vi "Data Viewer.vi"() -> ()   [LabVIEW 2018]
uses:
  Type/_Data.ctl
  <vilib>/Analysis/8numeric.llb/1D Numeric Integration.vi
  <vilib>/printing/ReportDocExtensions.llb/Append Front Panel Image to Report (path).vi
  <vilib>/Utility/NIReport.llb/NI_report.lvclass
  <vilib>/Utility/NIReport.llb/NI_ReportGenerationCore.lvlib
  <vilib>/Analysis/NI_AALPro.lvlib
  <vilib>/Analysis/NI_AALBase.lvlib
panel:
  out "File Name":string
  in  "Export 3":bool
  in  "Export 2":bool
  in  "Export":bool
  in  "Clear Last":bool
  in  "X scale to S":bool
  in  "Clear Offset":bool
  in  "Manual Offset":dbl format="%0.2f"
  in  "Subtract Manual":bool
  in  "Subtract File":bool
  in  "Subtract Mean":bool
  out "Mean":dbl format="%0.2f"
  out "Standard Deviation":dbl format="%0.2f"
  in  "Avg 4":bool caption="Avg"
  in  "Log 4":bool caption="Log"
  in  "CPS 4":bool caption="CPS"
  in  "Avg 3":bool caption="Avg"
  in  "Log 3":bool caption="Log"
  in  "CPS 3":bool caption="CPS"
  in  "Clear":bool
  in  "Add Overlay":bool
  out "Overlays":cluster{"X":sgl[], "Y":sgl[]}[](graph) caption="C:\\Users\\Tyler Doodeman\\Desktop\\April 5, 2018\\GC-C6\\722-GC-C6-5uL.isd; TIC=0; T=0mS"
  out "Integral":dbl format="%0.2f"
  out "TIC VS Time":cluster{"X":sgl[], "Y":sgl[]}(graph) caption="D:\\ProgrammsEI\\Sample#1 18_10_15_04_45PM.isd"
  out "XIC":cluster{"X":sgl[], "Y":sgl[]}(graph) caption="D:\\ProgrammsEI\\Sample#1 18_10_15_04_45PM.isd"
  in  "MR#":i32=1 caption="MR #"
  in  "Expt#":i32=1 caption="Expt #"
  in  "Scan#":i32=1 caption="Scan #"
  in  "Avg":bool
  in  "Log":bool
  in  "CPS":bool
  out "Spectrum":cluster{"X":sgl[], "Y":sgl[]}(graph) caption="D:\\ProgrammsEI\\Sample#1 18_10_15_04_45PM.isd; TIC=1; T=0mS"
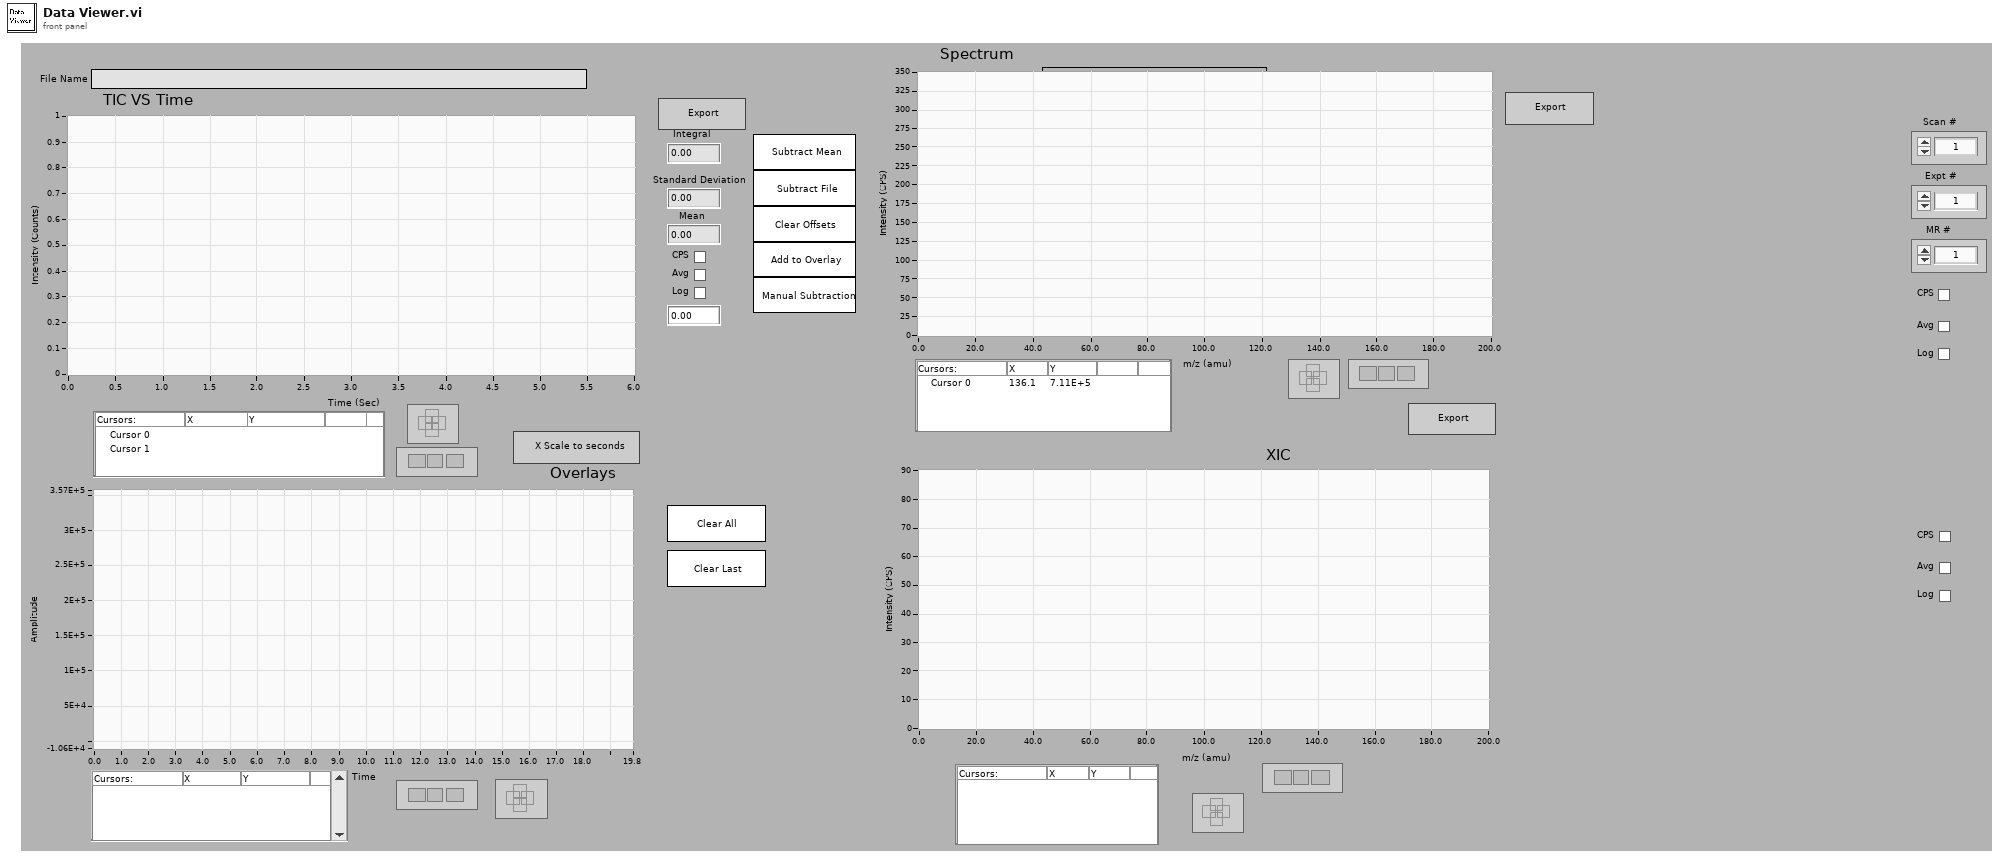
[diagram p1: front panel]
types:
  T1 = typedef "_Data.ctl" = cluster{"X":dbl[], "Y":dbl[], "Dwell Time (mS)":dbl, "X Title":string, "Time (s)":dbl, "TIC":u32, "# of Scans":i32, "Path":path, "ScanType":i32}
  T2 = cluster{"Spectrum Data":T1, "Spectrum":refnum<vi>, "TIC VS Time":refnum<vi>, "Path":path, "TIC Spectrum":refnum<vi>, "TIC VS Time Offset":dbl, "Overlay Offset":dbl, "XIC Data":T1, "Offset":dbl, "File Offset":dbl[], "Overlay Data":cluster{"X":sgl[], "Y":sgl[]}[], "TIC Spectrum":T1}
  T3 = enum32{"existing file", "new file", "new or existing file", "existing dir", "new dir", "new or existing dir", "existing file (use LLBs)", "new file (use LLBs)", "new or existing file (use LLBs)", "new or existing file or directory (use LLBs)"}
  T4 = enum16{"Standard Report", "HTML", "Word", "Excel"}
  T5 = typedef "imagedata.ctl" = cluster{"image type":i32, "image depth":i32, "image":u8[], "mask":u8[], "colors":u32[], "Rectangle":cluster{"left":i16, "top":i16, "right":i16, "bottom":i16}}
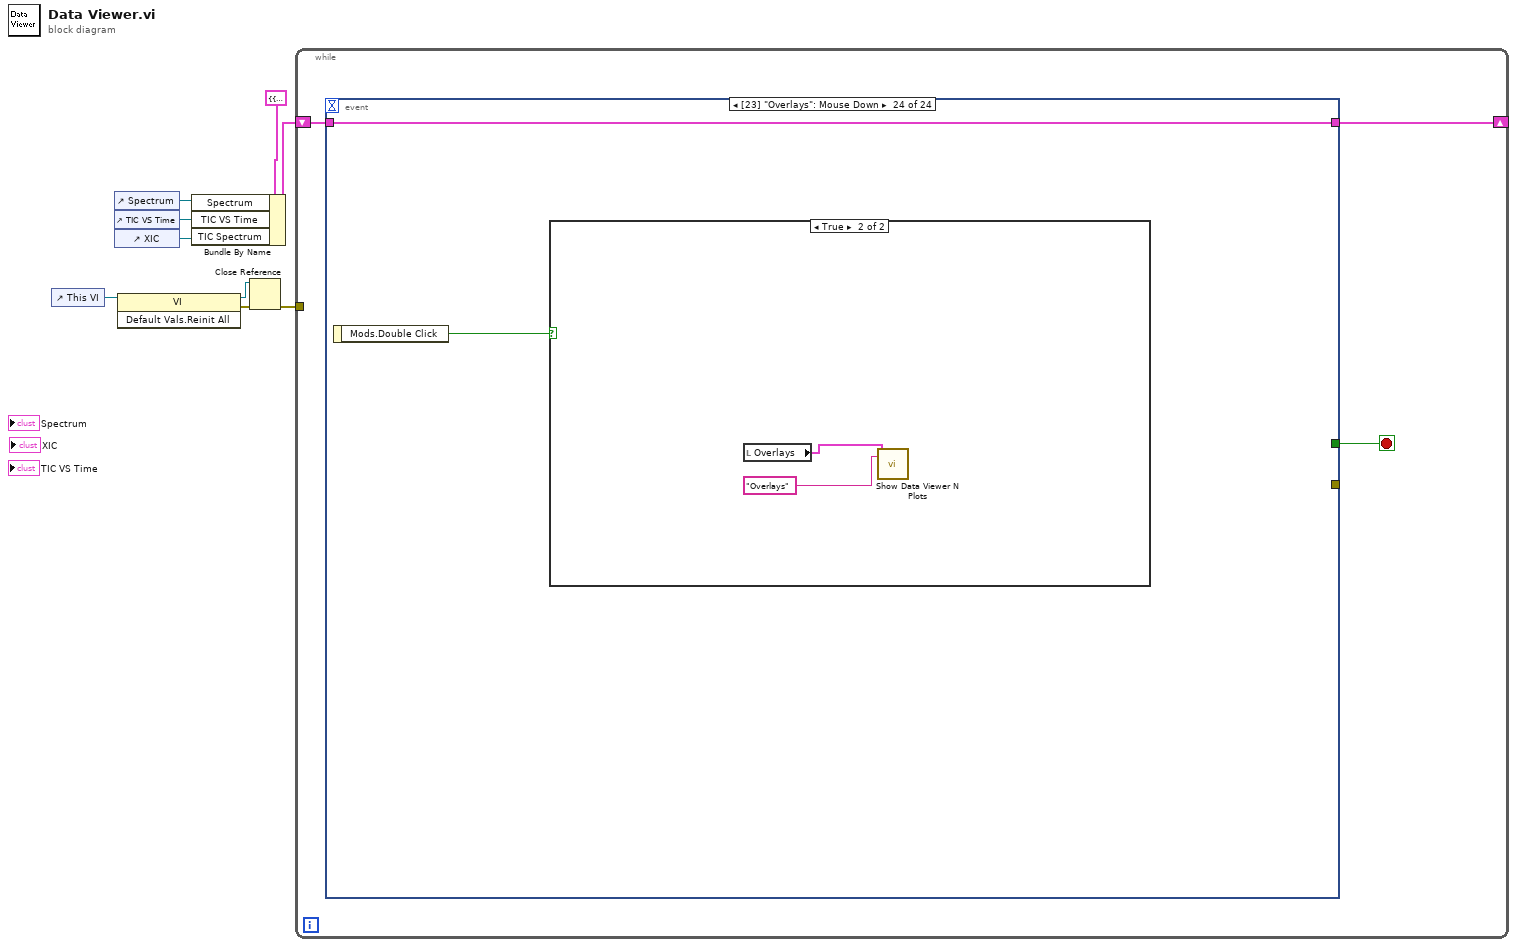
[diagram p0: block diagram]
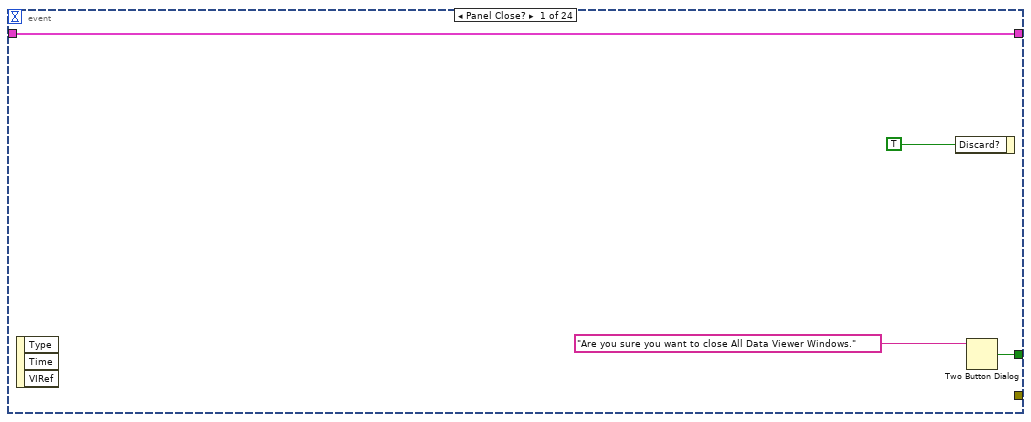
[diagram p2: hidden frame]
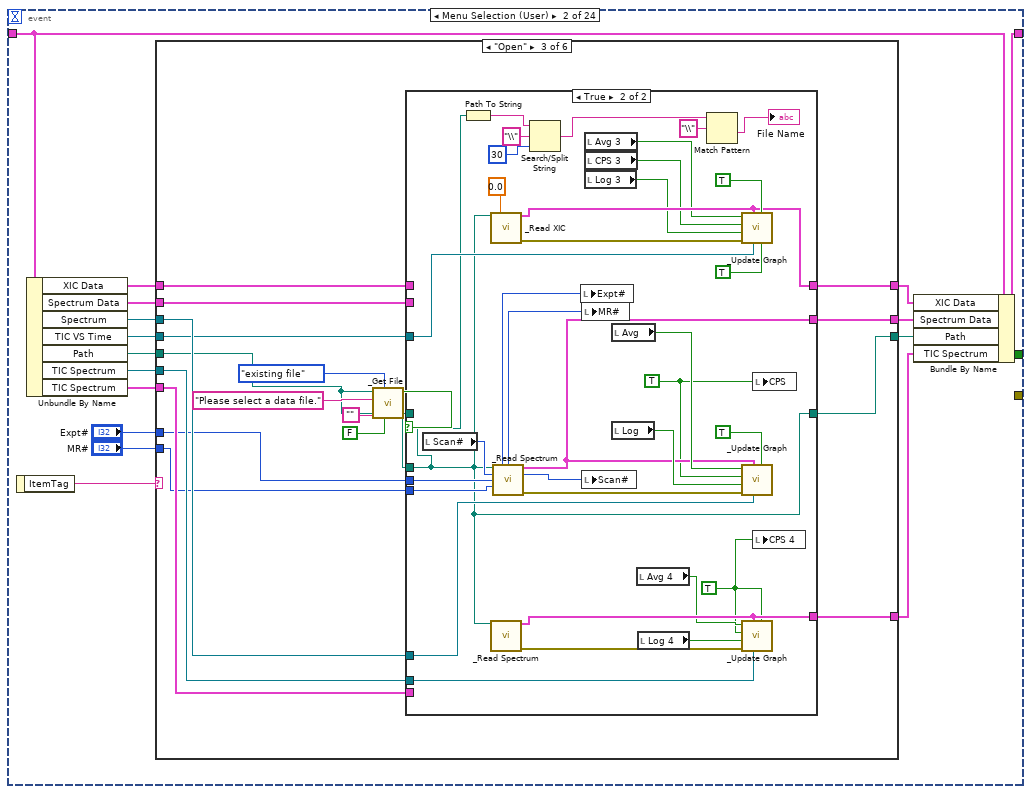
[diagram p3: hidden frame]
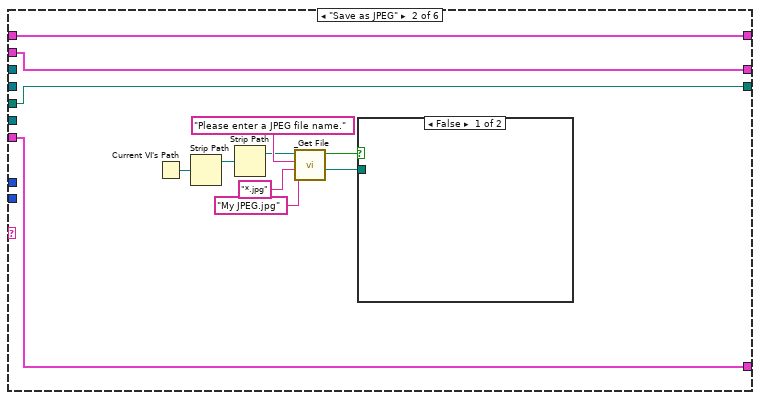
[diagram p5: hidden frame]
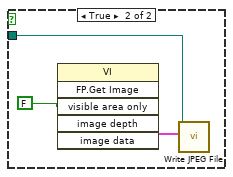
[diagram p6: hidden frame]
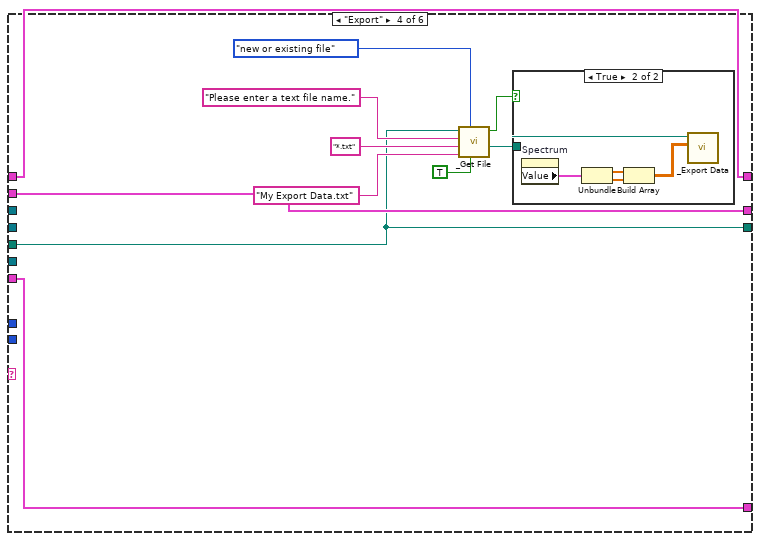
[diagram p8: hidden frame]
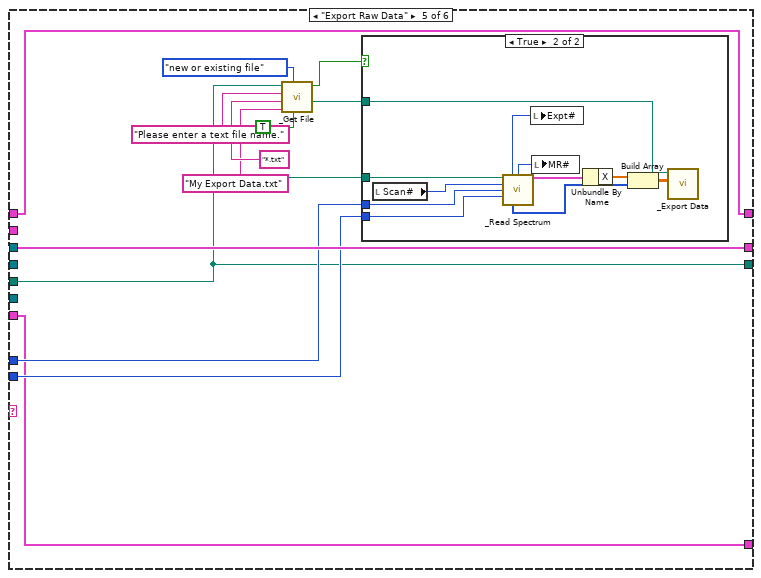
[diagram p10: hidden frame]
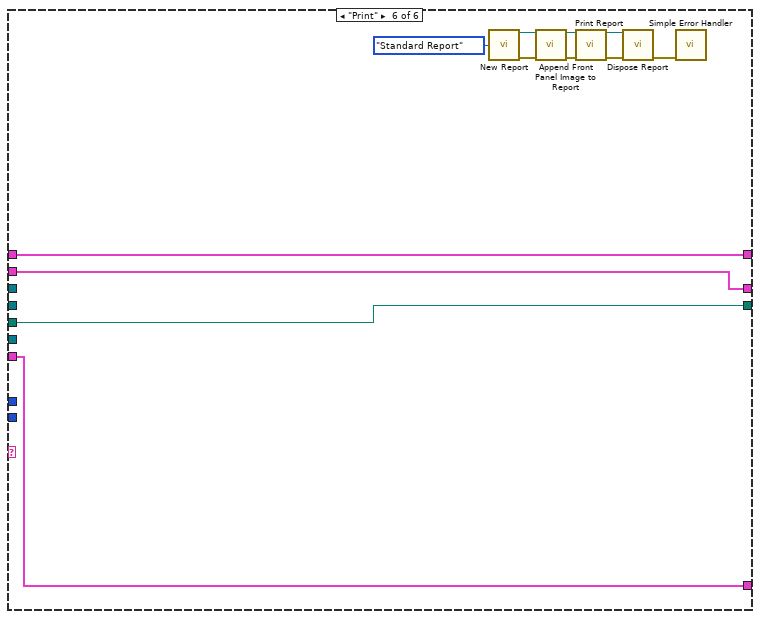
[diagram p12: hidden frame]
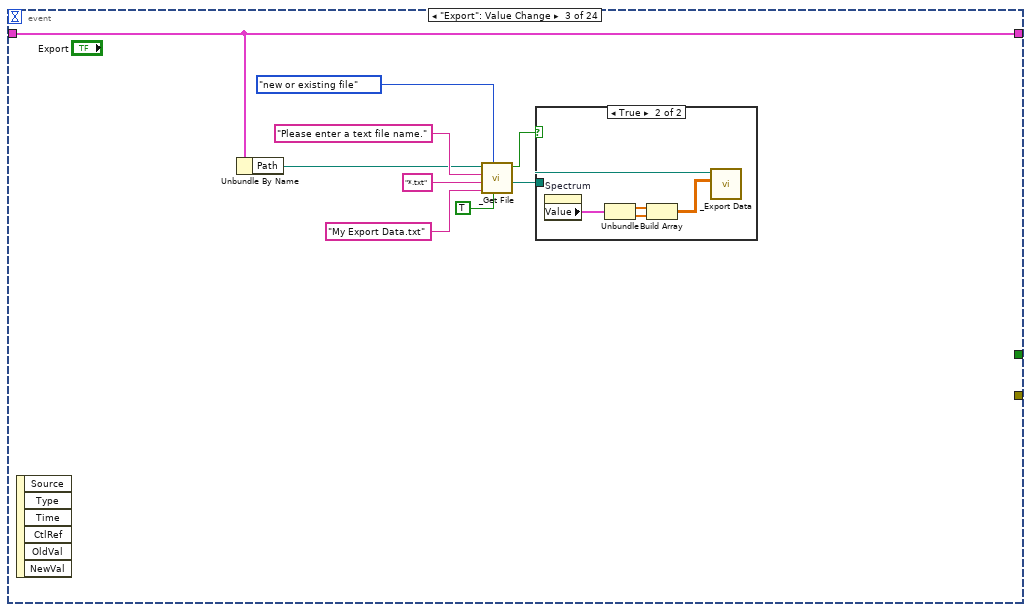
[diagram p13: hidden frame]
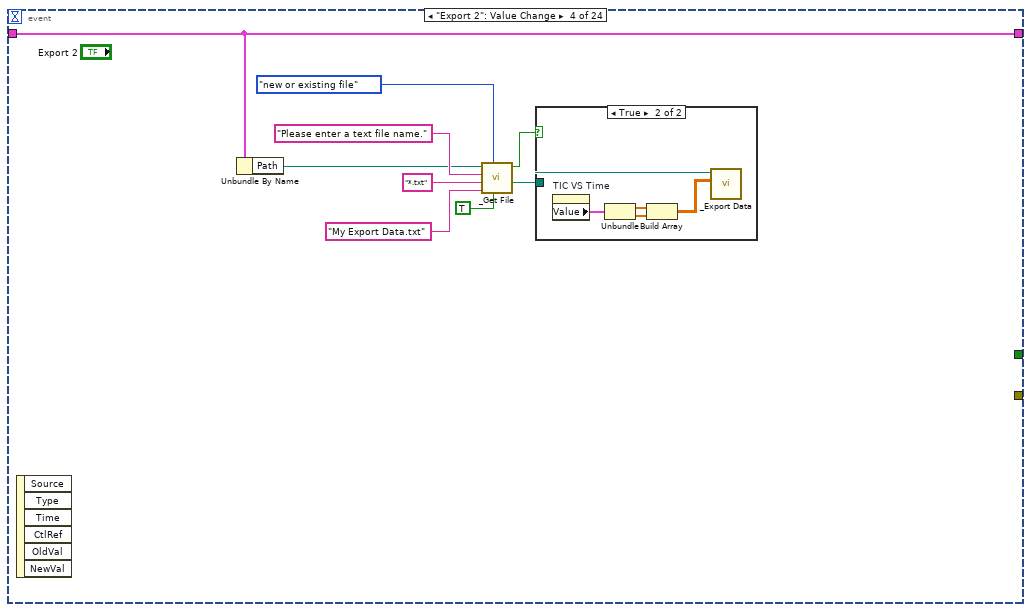
[diagram p15: hidden frame]
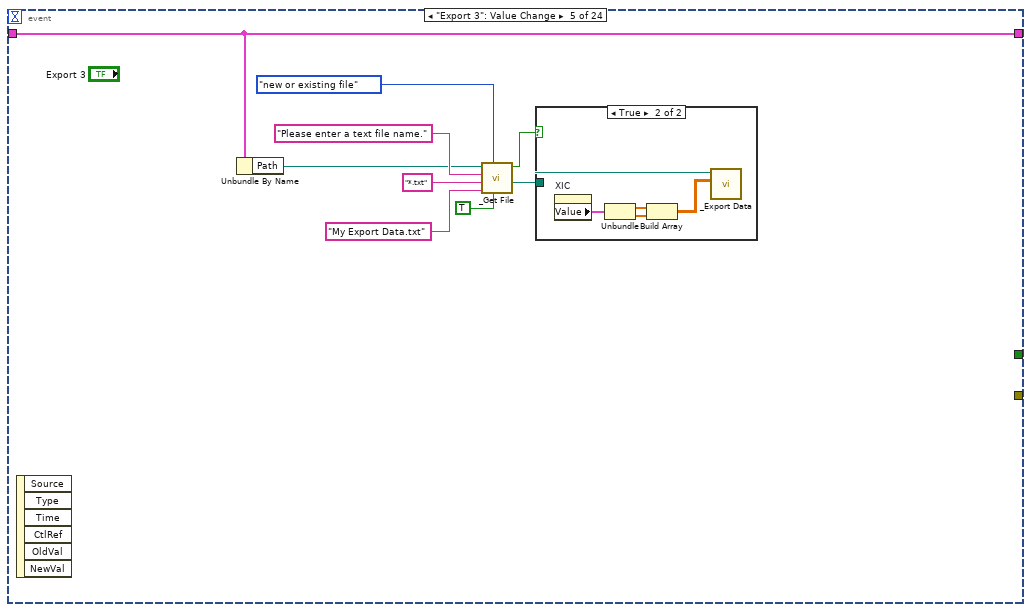
[diagram p17: hidden frame]
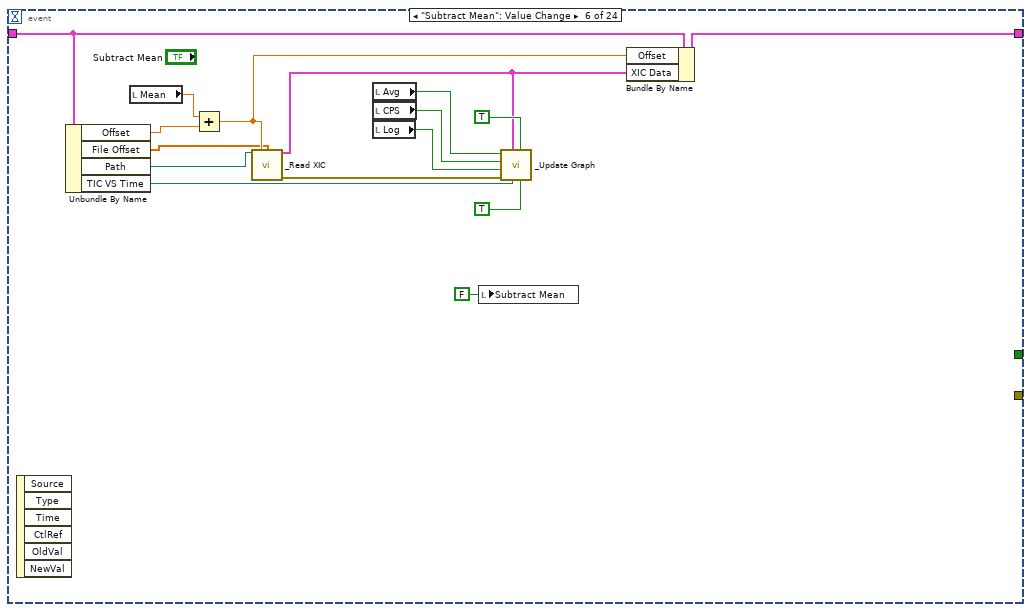
[diagram p19: hidden frame]
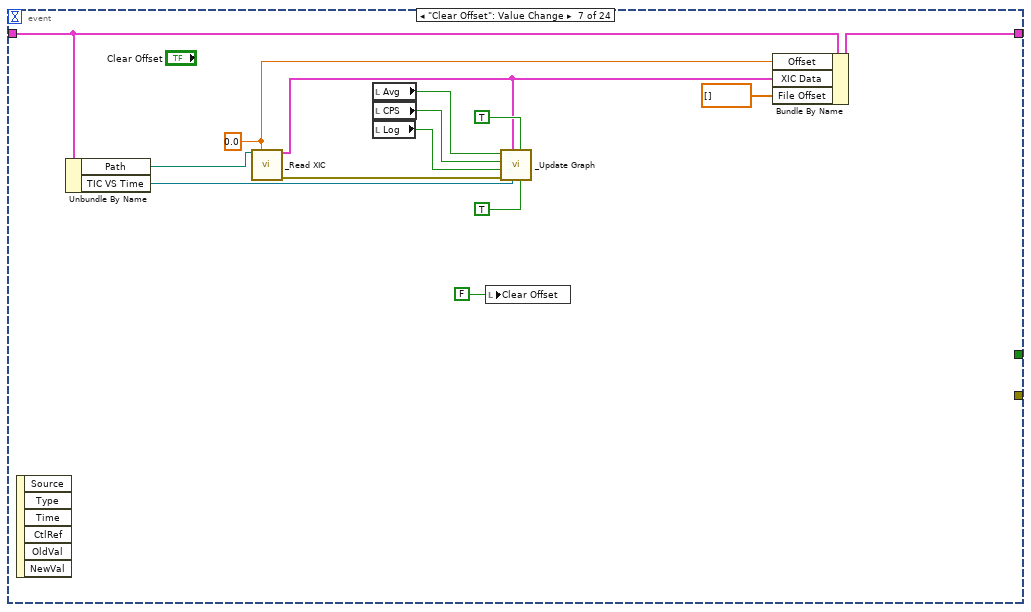
[diagram p20: hidden frame]
diagram:
  n1 = control-ref of="This VI"() -> (w4:refnum<vi>)
  n2 = control-ref of="Spectrum"() -> (w7:refnum<vi>)
  n3 = control-ref of="TIC VS Time"() -> (w6:refnum<vi>)
  n4 = control-ref of="XIC"() -> (w5:refnum<vi>)
  n5 = invoke class="VI" method="Default Vals.Reinit All"(reference=w4) -> (reference out=w2:refnum<vi>, error out=w3:errorcluster)  [unwired: 2 in, 1 out]
  n6 = Bundle By Name(cluster=T2 {"Spectrum Data"={"X"=[], "Y"=[], "Dwell Time (mS)"=0.0, "X Title"="", "Time (s)"=0.0, "TIC"=0, "# of Scans"=0, "Path"=path "", "ScanType"=0}, "Spectrum"=refnum, "TIC VS Time"=refnum, "Path"=path "", "TIC Spectrum"=refnum, "TIC VS Time Offset"=0.0, "Overlay Offset"=0.0, "XIC Data"={"X"=[], "Y"=[], "Dwell Time (mS)"=10.0, "X Title"="", "Time (s)"=0.0, "TIC"=0, "# of Scans"=133, "Path"=path "", "ScanType"=1}, "Offset"=0.0, "File Offset"=[], "Overlay Data"=[], "TIC Spectrum"={"X"=[], "Y"=[], "Dwell Time (mS)"=10.0, "X Title"="", "Time (s)"=0.0, "TIC"=0, "# of Scans"=133, "Path"=path "", "ScanType"=1}}, "Spectrum"=w7, "TIC VS Time"=w6, "TIC Spectrum"=w5) -> (w8:T2)
  n7 = Close Reference(reference=w2, error in (no error)=w3) -> (error out=w1:errorcluster)
  n8 = while {
    shift-right: [w10] -> _
    shift-left: w8 -> [w11]
    tunnel: w1 -> [_]
    stop <- w12 stop-if-true
    n9 = event shown="[23] \"Overlays\": Mouse Down" {
      selector: _ -> [_ _ _ _ _ _ _ _ _ _ _ _ _ _ _ _ _ _ _ _ _ _ _ _]
      dyn-events: _ -> [_ _ _ _ _ _ _ _ _ _ _ _ _ _ _ _ _ _ _ _ _ _ _ _]
      timeout: _ -> [_ _ _ _ _ _ _ _ _ _ _ _ _ _ _ _ _ _ _ _ _ _ _ _]
      tunnel: [w14 _ _ _ _ _ _ _ _ _ _ _ _ _ _ _ _ _ _ _ _ _ _ _] -> w12
      tunnel: w11 -> [w13 w26 w163 w177 w191 w213 w227 w243 w261 w283 w291 w299 w310 w318 w326 w345 w386 w399 w401 w405 w409 w414 w419 w424]
      tunnel: [w13 w25 w163 w177 w191 w210 w224 w240 w259 w281 w290 w299 w309 w318 w326 w344 w388 w399 w401 w405 w409 w414 w419 w424] -> w10
      tunnel: [_ _ _ _ _ _ _ _ _ _ w284 _ _ _ _ _ _ _ _ _ _ _ _ _] -> _
      event Panel Close? {
        n10 = event-data() -> ()  [unwired: 4 out]
        n11 = event-data("Discard?"=TRUE) -> ()  [unwired: 1 in, 1 out]
        n12 = Two Button Dialog(message="Are you sure you want to close All Data Viewer Windows.") -> (T button?=w14:bool)  [unwired: 2 out]
      }
      event Menu Selection (User) {
        n13 = event-data() -> ("ItemTag"=w32:string)  [unwired: 1 out]
        n14 = Unbundle By Name(w26) -> ("XIC Data"=w19:T1, "Spectrum Data"=w29:T1, "Spectrum"=w28:refnum<vi>, "TIC VS Time"=w27:refnum<vi>, "Path"=w22:path, "TIC Spectrum"=w21:refnum<vi>, "TIC Spectrum"=w17:T1)
        n15 = case shown="\"Open\"" w32 {
          tunnel: w29 -> [w36 w37 w66 w113 w131 w161]
          tunnel: [w36 w37 w65 w113 w131 w161] -> w24
          tunnel: w28 -> [_ _ w64 _ _ _]
          tunnel: "Expt#" -> [_ _ w53 _ w130 _]
          tunnel: "MR#" -> [_ _ w52 _ w129 _]
          tunnel: w27 -> [_ _ w62 _ _ _]
          tunnel: [w35 w48 w60 w112 w128 w152] -> w23
          tunnel: w22 -> [w35 w48 w59 w112 w128 w152]
          tunnel: w21 -> [_ _ w58 _ _ _]
          tunnel: [w34 w47 w57 w111 w127 w151] -> w20
          tunnel: w19 -> [w34 w47 w56 w111 w127 w151]
          tunnel: [w33 w46 w55 w110 w126 w150] -> w18
          tunnel: w17 -> [w33 w46 w54 w110 w126 w150]
          frame Default {
          }
          frame "Save as JPEG" {
            n16 = Current VI's Path() -> (path=w38:path)
            n17 = Strip Path(path=w38) -> (stripped path=w39:path)  [unwired: 1 out]
            n18 = Strip Path(path=w39) -> (stripped path=w40:path)  [unwired: 1 out]
            n19 = call "_Get File.vi"("default name"="My JPEG.jpg", "extension (isd)"="*.jpg", "prompt"="Please enter a JPEG file name.", "Start Path"=w40) -> ("Seleted File"=w45:path, "Succeeded"=w44:bool)  [unwired: 2 in, 2 out]
            n20 = case shown="False" w44 {
              tunnel: w45 -> [_ w49]
              frame False {
              }
              frame True {
                n21 = invoke class="VI" method="FP.Get Image"("visible area only"=FALSE ("Visible Area Only")) -> ("image data"=w50:T5)  [unwired: 5 in, 5 out]
                n22 = call <vilib>:"Write JPEG File.vi"("image data"=w50, "path to JPEG file"=w49) -> ()  [unwired: 1 in, 9 out]
              }
            }
          }
          frame "Open" {
            n23 = call "_Get File.vi"("For Write (T)"=FALSE, "select mode (new or existing)"=T3."existing file", "default name"="", "prompt"="Please select a data file.", "Start Path"=w59) -> ("Seleted File"=w61:path, "Succeeded"=w67:bool)  [unwired: 1 in, 2 out]
            n24 = case shown="True" w67 {
              tunnel: w61 -> [_ w88]
              tunnel: w66 -> [w74 _]
              tunnel: [w74 w105] -> w65
              tunnel: w64 -> [_ w104]
              tunnel: w62 -> [_ w96]
              tunnel: [w73 w88] -> w60
              tunnel: w59 -> [w73 _]
              tunnel: w58 -> [_ w95]
              tunnel: [w72 w93] -> w57
              tunnel: w56 -> [w72 _]
              tunnel: [w71 w92] -> w55
              tunnel: w54 -> [w71 _]
              tunnel: w53 -> [_ w91]
              tunnel: w52 -> [_ w90]
              frame False {
              }
              frame True {
                w87 = TRUE ("CPS")
                w82 = TRUE ("Auto Scale")
                n25 = local read "Scan#"() -> (w89:i32)
                n26 = Path To String(path=w88) -> (string=w80:string)
                n27 = call "_Read XIC.vi"("file path"=w88, "Offset"=0.0) -> ("Data"=w93:T1, "error out"=w99:errorcluster)  [unwired: 4 in, 8 out]
                n28 = call "_Read Spectrum.vi"("file path"=w88) -> ("Data"=w92:T1, "error out"=w97:errorcluster)  [unwired: 5 in, 8 out]
                n29 = call "_Read Spectrum.vi"("file path"=w88, "Scan# (1-based)"=w89, "Expt# (1-based)"=w91, "MR# (1-based)"=w90) -> ("Expt# Out"=w102:i32, "MR# Out"=w101:i32, "Data"=w105:T1, "Scan# out"=w109:i32, "error out"=w106:errorcluster)  [unwired: 2 in, 5 out]
                n30 = Search/Split String(string=w80, search string/char (-)="\\", offset (0)=30) -> (match + rest of string=w76:string)  [unwired: 2 out]
                n31 = local write "Expt#"(w102) -> ()
                n32 = local write "MR#"(w101) -> ()
                n33 = local write "Scan#"(w109) -> ()
                n34 = local read "Avg 3"() -> (w86:bool)
                n35 = local read "CPS 3"() -> (w85:bool)
                n36 = local read "Log 3"() -> (w84:bool)
                n37 = local read "Avg"() -> (w108:bool)
                n38 = local read "Log"() -> (w107:bool)
                n39 = local read "Avg 4"() -> (w83:bool)
                n40 = local read "Log 4"() -> (w81:bool)
                n41 = Match Pattern(string=w76, regular expression="\\") -> (after substring=→"File Name":string)  [unwired: 1 in, 3 out]
                n42 = call "_Update Graph.vi"("TIC (F)"=TRUE, "Auto Scale"=TRUE, "Graph Ref"=w96, "Data"=w93, "error in (no error)"=w99, "Log Scale"=w84, "CPS"=w85, "Averaging"=w86) -> ()  [unwired: 4 out]
                n43 = call "_Update Graph.vi"("Auto Scale"=TRUE, "Graph Ref"=w104, "Data"=w105, "error in (no error)"=w106, "Log Scale"=w107, "CPS"=w87, "Averaging"=w108) -> ()  [unwired: 1 in, 4 out]
                n44 = call "_Update Graph.vi"("Auto Scale"=w82, "Graph Ref"=w95, "Data"=w92, "error in (no error)"=w97, "Log Scale"=w81, "CPS"=w82, "Averaging"=w83) -> ()  [unwired: 1 in, 4 out]
                n45 = local write "CPS"(w87) -> ()
                n46 = local write "CPS 4"(w82) -> ()
              }
            }
          }
          frame "Export" {
            n47 = call "_Get File.vi"("For Write (T)"=TRUE, "select mode (new or existing)"=T3."new or existing file", "default name"="My Export Data.txt", "extension (isd)"="*.txt", "prompt"="Please enter a text file name.", "Start Path"=w112) -> ("Seleted File"=w116:path, "Succeeded"=w117:bool)  [unwired: 2 out]
            n48 = case shown="True" w117 {
              tunnel: w116 -> [_ w125]
              frame False {
              }
              frame True {
                n49 = property on="Spectrum" class="XYGraph (strict)"() -> ("Value"=w123:cluster{"X":sgl[], "Y":sgl[]})  [unwired: 2 in, 2 out]
                n50 = Unbundle(w123) -> ("X"=w122:sgl[], "Y"=w121:sgl[])
                n51 = Build Array(w122, w121) -> (w124:sgl[][])
                n52 = call "_Export Data.vi"("2D data"=w124, "file path (dialog if empty)"=w125) -> ()  [unwired: 1 in, 6 out]
              }
            }
          }
          frame "Export Raw Data" {
            n53 = call "_Get File.vi"("For Write (T)"=TRUE, "select mode (new or existing)"=T3."new or existing file", "default name"="My Export Data.txt", "extension (isd)"="*.txt", "prompt"="Please enter a text file name.", "Start Path"=w128) -> ("Seleted File"=w134:path, "Succeeded"=w135:bool)  [unwired: 2 out]
            n54 = case shown="True" w135 {
              tunnel: w134 -> [_ w149]
              tunnel: w130 -> [_ w143]
              tunnel: w129 -> [_ w141]
              tunnel: w128 -> [_ w139]
              frame False {
              }
              frame True {
                n55 = local read "Scan#"() -> (w147:i32)
                n56 = call "_Read Spectrum.vi"("file path"=w139, "Scan# (1-based)"=w147, "Expt# (1-based)"=w143, "MR# (1-based)"=w141) -> ("Expt# Out"=w142:i32, "MR# Out"=w140:i32, "Data"=w146:T1, "raw data"=w144:i32[])  [unwired: 2 in, 6 out]
                n57 = local write "Expt#"(w142) -> ()
                n58 = local write "MR#"(w140) -> ()
                n59 = Unbundle By Name(w146) -> ("X"=w145:dbl[])
                n60 = Build Array(w145, w144) -> (w148:dbl[][])
                n61 = call "_Export Data.vi"("2D data"=w148, "file path (dialog if empty)"=w149) -> ()  [unwired: 1 in, 6 out]
              }
            }
          }
          frame "Print" {
            n62 = call <vilib>:"New Report.vi"("report type"=T4."Standard Report") -> ("report out"=w157:refnum<class "NI_report.lvclass">, "error out"=w158:errorcluster)  [unwired: 5 in, 8 out]
            n63 = call-poly <vilib>:"Append Front Panel Image to Report.vi"("report in"=w157, "error in (no error)"=w158) -> ("report out"=w159:refnum<class "NI_report.lvclass">, "error out"=w160:errorcluster)  [unwired: 6 in, 6 out]
            n64 = call-dynamic "Print Report.vi"("report in"=w159, "error in (no error)"=w160) -> ("report out"=w155:refnum<class "NI_report.lvclass">, "error out"=w156:errorcluster)  [unwired: 2 in, 10 out]
            n65 = call-dynamic "Dispose Report.vi"("report in"=w155, "error in (no error)"=w156) -> ("error out"=w154:errorcluster)  [unwired: 3 in, 10 out]
            n66 = call <vilib>:"Simple Error Handler.vi"("error in (no error)"=w154) -> ()  [unwired: 1 in, 8 out]
          }
        }
        n67 = Bundle By Name(cluster=w26, "XIC Data"=w20, "Spectrum Data"=w24, "Path"=w23, "TIC Spectrum"=w18) -> (w25:T2)
      }
      event "Export": Value Change {
        n68 = event-data() -> ()  [unwired: 7 out]
        n69 = Unbundle By Name(w163) -> ("Path"=w162:path)
        n70 = call "_Get File.vi"("For Write (T)"=TRUE, "select mode (new or existing)"=T3."new or existing file", "default name"="My Export Data.txt", "extension (isd)"="*.txt", "prompt"="Please enter a text file name.", "Start Path"=w162) -> ("Seleted File"=w168:path, "Succeeded"=w167:bool)  [unwired: 2 out]
        n71 = case shown="True" w167 {
          tunnel: w168 -> [_ w175]
          frame False {
          }
          frame True {
            n72 = property on="Spectrum" class="XYGraph (strict)"() -> ("Value"=w173:cluster{"X":sgl[], "Y":sgl[]})  [unwired: 2 in, 2 out]
            n73 = Unbundle(w173) -> ("X"=w172:sgl[], "Y"=w171:sgl[])
            n74 = Build Array(w172, w171) -> (w174:sgl[][])
            n75 = call "_Export Data.vi"("2D data"=w174, "file path (dialog if empty)"=w175) -> ()  [unwired: 1 in, 6 out]
          }
        }
      }
      event "Export 2": Value Change {
        n76 = event-data() -> ()  [unwired: 7 out]
        n77 = Unbundle By Name(w177) -> ("Path"=w176:path)
        n78 = call "_Get File.vi"("For Write (T)"=TRUE, "select mode (new or existing)"=T3."new or existing file", "default name"="My Export Data.txt", "extension (isd)"="*.txt", "prompt"="Please enter a text file name.", "Start Path"=w176) -> ("Seleted File"=w182:path, "Succeeded"=w181:bool)  [unwired: 2 out]
        n79 = case shown="True" w181 {
          tunnel: w182 -> [_ w189]
          frame False {
          }
          frame True {
            n80 = property on="TIC VS Time" class="XYGraph (strict)"() -> ("Value"=w187:cluster{"X":sgl[], "Y":sgl[]})  [unwired: 2 in, 2 out]
            n81 = Unbundle(w187) -> ("X"=w186:sgl[], "Y"=w185:sgl[])
            n82 = Build Array(w186, w185) -> (w188:sgl[][])
            n83 = call "_Export Data.vi"("2D data"=w188, "file path (dialog if empty)"=w189) -> ()  [unwired: 1 in, 6 out]
          }
        }
      }
      event "Export 3": Value Change {
        n84 = event-data() -> ()  [unwired: 7 out]
        n85 = Unbundle By Name(w191) -> ("Path"=w190:path)
        n86 = call "_Get File.vi"("For Write (T)"=TRUE, "select mode (new or existing)"=T3."new or existing file", "default name"="My Export Data.txt", "extension (isd)"="*.txt", "prompt"="Please enter a text file name.", "Start Path"=w190) -> ("Seleted File"=w196:path, "Succeeded"=w195:bool)  [unwired: 2 out]
        n87 = case shown="True" w195 {
          tunnel: w196 -> [_ w203]
          frame False {
          }
          frame True {
            n88 = property on="XIC" class="XYGraph (strict)"() -> ("Value"=w201:cluster{"X":sgl[], "Y":sgl[]})  [unwired: 2 in, 2 out]
            n89 = Unbundle(w201) -> ("X"=w200:sgl[], "Y"=w199:sgl[])
            n90 = Build Array(w200, w199) -> (w202:sgl[][])
            n91 = call "_Export Data.vi"("2D data"=w202, "file path (dialog if empty)"=w203) -> ()  [unwired: 1 in, 6 out]
          }
        }
      }
      event "Subtract Mean": Value Change {
        n92 = event-data() -> ()  [unwired: 7 out]
        n93 = Unbundle By Name(w213) -> ("Offset"=w208:dbl, "File Offset"=w204:dbl[], "Path"=w211:path, "TIC VS Time"=w212:refnum<vi>)
        n94 = local read "Mean"() -> (w207:dbl)
        n95 = Add(x=w207, y=w208) -> (x+y=w206:dbl)
        n96 = call "_Read XIC.vi"("file path"=w211, "Offset"=w206, "File Offset"=w204) -> ("Data"=w209:T1, "error out"=w215:errorcluster)  [unwired: 3 in, 8 out]
        n97 = local read "Avg"() -> (w219:bool)
        n98 = local read "CPS"() -> (w218:bool)
        n99 = local read "Log"() -> (w217:bool)
        n100 = local write "Subtract Mean"(FALSE ("Subtract Mean")) -> ()
        n101 = call "_Update Graph.vi"("TIC (F)"=TRUE, "Auto Scale"=TRUE, "Graph Ref"=w212, "Data"=w209, "error in (no error)"=w215, "Log Scale"=w217, "CPS"=w218, "Averaging"=w219) -> ()  [unwired: 4 out]
        n102 = Bundle By Name(cluster=w213, "Offset"=w206, "XIC Data"=w209) -> (w210:T2)
      }
      event "Clear Offset": Value Change {
        w221 = 0.0 ("Offset")
        n103 = event-data() -> ()  [unwired: 7 out]
        n104 = Unbundle By Name(w227) -> ("Path"=w225:path, "TIC VS Time"=w226:refnum<vi>)
        n105 = call "_Read XIC.vi"("file path"=w225, "Offset"=w221) -> ("Data"=w223:T1, "error out"=w229:errorcluster)  [unwired: 4 in, 8 out]
        n106 = local read "Avg"() -> (w233:bool)
        n107 = local read "CPS"() -> (w232:bool)
        n108 = local read "Log"() -> (w231:bool)
        n109 = local write "Clear Offset"(FALSE ("Subtract Mean")) -> ()
        n110 = call "_Update Graph.vi"("TIC (F)"=TRUE, "Auto Scale"=TRUE, "Graph Ref"=w226, "Data"=w223, "error in (no error)"=w229, "Log Scale"=w231, "CPS"=w232, "Averaging"=w233) -> ()  [unwired: 4 out]
        n111 = Bundle By Name(cluster=w227, "Offset"=w221, "XIC Data"=w223, "File Offset"=dbl[] []) -> (w224:T2)
      }
      event "Subtract Manual": Value Change {
        n112 = event-data() -> ()  [unwired: 7 out]
        n113 = Unbundle By Name(w243) -> ("Offset"=w238:dbl, "File Offset"=w235:dbl[], "Path"=w241:path, "TIC VS Time"=w242:refnum<vi>)
        n114 = Add(x="Manual Offset", y=w238) -> (x+y=w237:dbl)
        n115 = call "_Read XIC.vi"("file path"=w241, "Offset"=w237, "File Offset"=w235) -> ("Data"=w239:T1, "error out"=w245:errorcluster)  [unwired: 3 in, 8 out]
        n116 = local read "Avg"() -> (w249:bool)
        n117 = local read "CPS"() -> (w248:bool)
        n118 = local read "Log"() -> (w247:bool)
        n119 = call "_Update Graph.vi"("TIC (F)"=TRUE, "Auto Scale"=TRUE, "Graph Ref"=w242, "Data"=w239, "error in (no error)"=w245, "Log Scale"=w247, "CPS"=w248, "Averaging"=w249) -> ()  [unwired: 4 out]
        n120 = local write "Subtract Manual"(FALSE ("Subtract Manual")) -> ()
        n121 = Bundle By Name(cluster=w243, "Offset"=w237, "Spectrum Data"=w239) -> (w240:T2)
      }
      event "Subtract File": Value Change {
        n122 = event-data() -> ()  [unwired: 7 out]
        n123 = Unbundle By Name(w261) -> ("Offset"=w258:dbl, "Path"=w252:path, "TIC VS Time"=w260:refnum<vi>)
        n124 = call "_Get File.vi"("For Write (T)"=FALSE, "select mode (new or existing)"=T3."existing file", "default name"="", "prompt"="Please select a data file.", "Start Path"=w252) -> ("Seleted File"=w251:path, "Succeeded"=w250:bool)  [unwired: 1 in, 2 out]
        n125 = case shown="True" w250 {
          tunnel: w261 -> [w262 w272]
          tunnel: w260 -> [_ w271]
          tunnel: [w262 w270] -> w259
          tunnel: w258 -> [_ w268]
          tunnel: w252 -> [_ w267]
          tunnel: w251 -> [_ w266]
          frame False {
          }
          frame True {
            n126 = call "_Read XIC.vi"("file path"=w266, "Offset"=0.0) -> ("Data"=w265:T1)  [unwired: 4 in, 9 out]
            n127 = Unbundle By Name(w265) -> ("Y"=w264:dbl[])
            n128 = call "_Read XIC.vi"("file path"=w267, "Offset"=w268, "File Offset"=w264) -> ("Data"=w269:T1, "error out"=w274:errorcluster)  [unwired: 3 in, 8 out]
            n129 = local read "Avg"() -> (w278:bool)
            n130 = local read "CPS"() -> (w277:bool)
            n131 = local read "Log"() -> (w276:bool)
            n132 = call "_Update Graph.vi"("TIC (F)"=TRUE, "Auto Scale"=TRUE, "Graph Ref"=w271, "Data"=w269, "error in (no error)"=w274, "Log Scale"=w276, "CPS"=w277, "Averaging"=w278) -> ()  [unwired: 4 out]
            n133 = Bundle By Name(cluster=w272, "XIC Data"=w269, "File Offset"=w264) -> (w270:T2)
          }
        }
        n134 = local write "Subtract File"(FALSE ("Subtract Manual")) -> ()
      }
      event "Add Overlay": Value Change {
        n135 = event-data() -> ()  [unwired: 7 out]
        n136 = Unbundle By Name(w283) -> ("Overlay Data"=w282:cluster{"X":sgl[], "Y":sgl[]}[])
        n137 = local read "TIC VS Time"() -> (w280:cluster{"X":sgl[], "Y":sgl[]})
        n138 = Build Array (concatenate)(w282, w280) -> (w279:cluster{"X":sgl[], "Y":sgl[]}[])
        n139 = Bundle By Name(cluster=w283, "Overlay Data"=w279) -> (w281:T2)
        n140 = property on="Overlays" class="XYGraph (strict)"("Value"=w279) -> ()  [unwired: 2 in, 2 out]
      }
      event "Clear Last": Value Change {
        n141 = event-data() -> ()  [unwired: 7 out]
        n142 = Unbundle By Name(w291) -> ("Overlay Data"=w287:cluster{"X":sgl[], "Y":sgl[]}[])
        n143 = Array Size(array=w287) -> (size(s)=w286:i32)
        n144 = Decrement(x=w286) -> (x-1=w285:i32)
        n145 = Delete From Array(array=w287, length=1, index=w285) -> (array with subset deleted=w289:cluster{"X":sgl[], "Y":sgl[]}[])  [unwired: 1 out]
        n146 = Bundle By Name(cluster=w291, "Overlay Data"=w289) -> (w290:T2)
        n147 = property on="Overlays" class="XYGraph (strict)"("Value"=w289) -> (error out=w284:errorcluster)  [unwired: 2 in, 1 out]
      }
      event "X scale to S": Value Change {
        n148 = event-data() -> ("NewVal"=w293:bool)  [unwired: 1 out]
        n149 = local read "TIC VS Time"() -> (w296:cluster{"X":sgl[], "Y":sgl[]})
        n150 = Unbundle By Name(w296) -> ("X"=w298:sgl[])
        n151 = case shown="True" w293 {
          tunnel: w298 -> [w303 w307]
          tunnel: 60.0 -> [w302 w306]
          tunnel: [w301 w305] -> w295
          tunnel: ["Time (Sec)" ("X Scale.Name Label.Text") "Time (Min)" ("X Scale.Name Label.Text")] -> w292
          frame True {
            n152 = Multiply(x=w303, y=w302) -> (x*y=w301:dbl[])
          }
          frame False {
            n153 = Divide(x=w307, y=w306) -> (x/y=w305:dbl[])
          }
        }
        n154 = Bundle By Name(cluster=w296, "X"=w295) -> (w294:cluster{"X":sgl[], "Y":sgl[]})
        n155 = property on="TIC VS Time" class="XYGraph (strict)"("Value"=w294, "XScale.NameLbl.Text"=w292) -> ()  [unwired: 2 in, 2 out]
      }
      event "Clear": Value Change {
        w308 = cluster{"X":sgl[], "Y":sgl[]}[] [] ("Overlay Data")
        n156 = event-data() -> ()  [unwired: 7 out]
        n157 = Bundle By Name(cluster=w310, "Overlay Data"=w308) -> (w309:T2)
        "Overlays" <- w308
      }
      event "CPS 3", "Log 3", "Avg 3": Value Change {
        n158 = event-data() -> ()  [unwired: 7 out]
        n159 = Unbundle By Name(w318) -> ("XIC Data"=w317:T1, "TIC VS Time"=w316:refnum<vi>)
        n160 = call "_Update Graph.vi"("TIC (F)"=TRUE, "Auto Scale"=TRUE, "Graph Ref"=w316, "Data"=w317, "Log Scale"="Log 3", "CPS"="CPS 3", "Averaging"="Avg 3") -> ()  [unwired: 1 in, 4 out]
      }
      event "CPS 4", "Log 4", "Avg 4": Value Change {
        n161 = event-data() -> ()  [unwired: 7 out]
        n162 = Unbundle By Name(w326) -> ("TIC Spectrum"=w325:T1, "TIC Spectrum"=w324:refnum<vi>)
        n163 = call "_Update Graph.vi"("TIC (F)"=TRUE, "Auto Scale"=TRUE, "Graph Ref"=w324, "Data"=w325, "Log Scale"="Log 4", "CPS"="CPS 4", "Averaging"="Avg 4") -> ()  [unwired: 1 in, 4 out]
      }
      event "TIC VS Time": Cursor Move {
        n164 = event-data() -> ("PointIdx"=w367:i32)  [unwired: 1 out]
        n165 = for {
          N: 2 -> [_]
          tunnel: [w382] -> w363 mode=indexing
          i -> [w383]
          n166 = property on="TIC VS Time" class="XYGraph (strict)"("Active Cursor"=w383) -> ("Cursor.Cursor Index"=w382:i32)  [unwired: 2 in, 2 out]
        }
        n167 = Sort 1D Array(array=w363) -> (sorted array=w342:i32[])
        n168 = Increment(x=w342) -> (x+1=w337:i32[])
        n169 = Increment(x=w367) -> (x+1=w366:i32)
        n170 = Unbundle By Name(w345) -> ("Path"=w343:path)
        n171 = Index Array(array=w337, index #1=1 ("index"), index #2=0 ("index")) -> (element #1=w339:i32, element #2=w336:i32)
        n172 = property on="TIC VS Time" class="XYGraph (strict)"() -> ("Value"=w359:cluster{"X":sgl[], "Y":sgl[]})  [unwired: 2 in, 2 out]
        n173 = Subtract(x=w339, y=w336) -> (x-y=w338:i32)
        n174 = Unbundle By Name(w359) -> ("X"=w355:sgl[], "Y"=w358:sgl[])
        n175 = call "_Read Spectrum.vi"("file path"=w343, "Scan# (1-based)"=w366) -> ("Data"=w332:T1, "error out"=w329:errorcluster)  [unwired: 4 in, 8 out]
        n176 = Index Array(array=w342, index #1=1 ("index"), index #2=0 ("index")) -> (element #1=w360:i32, element #2=w356:i32)
        n177 = Unbundle By Name(w332) -> ("X"=w335:dbl[])
        n178 = Subtract(x=w360, y=w356) -> (x-y=w357:i32)
        n179 = Index Array(array=w355, index #1=1 ("index"), index #2=0 ("index")) -> (element #1=w352:sgl, element #2=w351:sgl)
        n180 = Array Size(array=w335) -> (size(s)=w327:i32)
        n181 = Initialize Array(0.0 ("element"), w327) -> (w333:dbl[])
        n182 = for {
          N: w338 -> [_]
          tunnel: w343 -> [w381]
          tunnel: w336 -> [w378]
          shift-right: [w375] -> w330
          shift-left: w333 -> [w374]
          shift-right: [w372] -> w328
          shift-left: w329 -> [w373]
          i -> [w380]
          n183 = Add(x=w378, y=w380) -> (x+y=w379:i32)
          n184 = call "_Read Spectrum.vi"("file path"=w381, "Scan# (1-based)"=w379, "error in (no error)"=w373) -> ("Data"=w377:T1, "error out"=w372:errorcluster)  [unwired: 3 in, 8 out]
          n185 = Unbundle By Name(w377) -> ("Y"=w376:dbl[])
          n186 = Add(x=w376, y=w374) -> (x+y=w375:dbl[])
        }
        n187 = Subtract(x=w352, y=w351) -> (x-y=w350:sgl)
        n188 = Array Subset(array=w358, index=w356, length=w357) -> (w348:sgl[])
        n189 = call-poly <vilib>:"Numeric Integration.vi"("dt"=w350, "Input Array"=w348) -> ("result"=→"Integral":dbl)  [unwired: 1 in, 1 out]
        n190 = call <vilib>:"Std Deviation and Variance.vi"("X"=w348) -> ("mean"=→"Mean":dbl, "standard deviation"=→"Standard Deviation":dbl)  [unwired: 1 in, 1 out]
        n191 = Bundle By Name(cluster=w332, "Y"=w330) -> (w331:T1)
        n192 = Bundle By Name(cluster=w345, "TIC Spectrum"=w332) -> (w344:T2)
        n193 = local read "Avg"() -> (w371:bool)
        n194 = local read "CPS"() -> (w370:bool)
        n195 = local read "Log"() -> (w369:bool)
        n196 = control-ref of="XIC"() -> (w365:refnum<vi>)
        n197 = call "_Update Graph.vi"("Auto Scale"=TRUE, "Graph Ref"=w365, "Data"=w331, "error in (no error)"=w328, "Log Scale"=w369, "CPS"=w370, "Averaging"=w371) -> ()  [unwired: 1 in, 4 out]
      }
      event "Scan#": Value Change {
        n198 = event-data() -> ("NewVal"=w393:i32)  [unwired: 1 out]
        n199 = Unbundle By Name(w386) -> ("Path"=w384:path, "Spectrum"=w385:refnum<vi>)
        n200 = local read "Expt#"() -> (w391:i32)
        n201 = local read "MR#"() -> (w390:i32)
        n202 = call "_Read Spectrum.vi"("file path"=w384, "Scan# (1-based)"=w393, "Expt# (1-based)"=w391, "MR# (1-based)"=w390) -> ("Expt# Out"=w392:i32, "MR# Out"=w389:i32, "Data"=w387:T1, "Scan# out"=w398:i32, "error out"=w394:errorcluster)  [unwired: 2 in, 5 out]
        n203 = local write "Expt#"(w392) -> ()
        n204 = local write "MR#"(w389) -> ()
        n205 = local write "Scan#"(w398) -> ()
        n206 = local read "Avg"() -> (w397:bool)
        n207 = local read "CPS"() -> (w396:bool)
        n208 = local read "Log"() -> (w395:bool)
        n209 = Bundle By Name(cluster=w386, "Spectrum Data"=w387) -> (w388:T2)
        n210 = call "_Update Graph.vi"("Graph Ref"=w385, "Data"=w387, "error in (no error)"=w394, "Log Scale"=w395, "CPS"=w396, "Averaging"=w397) -> ()  [unwired: 2 in, 4 out]
      }
      event "Expt#": Value Change {
        n211 = event-data() -> ()  [unwired: 2 out]
        n212 = property on="Scan#" class="DigNum (strict)"("Val(Sgnl)"="Scan#") -> ()  [unwired: 2 in, 2 out]
      }
      event "MR#": Value Change {
        n213 = event-data() -> ()  [unwired: 2 out]
        n214 = local read "Scan#"() -> (w402:i32)
        n215 = property on="Scan#" class="DigNum (strict)"("Val(Sgnl)"=w402) -> ()  [unwired: 2 in, 2 out]
      }
      event "CPS", "Log", "Avg": Value Change {
        n216 = event-data() -> ()  [unwired: 7 out]
        n217 = Unbundle By Name(w405) -> ("Spectrum Data"=w404:T1, "Spectrum"=w403:refnum<vi>)
        n218 = call "_Update Graph.vi"("Graph Ref"=w403, "Data"=w404, "Log Scale"="Log", "CPS"="CPS", "Averaging"="Avg") -> ()  [unwired: 3 in, 4 out]
      }
      event "Spectrum": Mouse Down {
        n219 = event-data() -> ("Mods.Double Click"=w410:bool)  [unwired: 1 out]
        n220 = case shown="True" w410 {
          frame False {
          }
          frame True {
            n221 = property on="Spectrum" class="XYGraph (strict)"() -> ("Value"=w412:cluster{"X":sgl[], "Y":sgl[]}, "YScale.NameLbl.Text"=w411:string)  [unwired: 2 in, 2 out]
            n222 = call "Show Data Viewer Plot.vi"("Caption.Text"="Spectrum", "Y Scale.Unit Label.Text"=w411, "Graph"=w412) -> ()  [unwired: 9 in]
          }
        }
      }
      event "TIC VS Time": Mouse Down {
        n223 = event-data() -> ("Mods.Double Click"=w415:bool)  [unwired: 1 out]
        n224 = case shown="True" w415 {
          frame False {
          }
          frame True {
            n225 = property on="TIC VS Time" class="XYGraph (strict)"() -> ("Value"=w417:cluster{"X":sgl[], "Y":sgl[]}, "YScale.NameLbl.Text"=w416:string)  [unwired: 2 in, 2 out]
            n226 = call "Show Data Viewer Plot.vi"("Caption.Text"="TIC VS Time", "Y Scale.Unit Label.Text"=w416, "Graph"=w417) -> ()  [unwired: 9 in]
          }
        }
      }
      event "XIC": Mouse Down {
        n227 = event-data() -> ("Mods.Double Click"=w420:bool)  [unwired: 1 out]
        n228 = case shown="True" w420 {
          frame False {
          }
          frame True {
            n229 = property on="XIC" class="XYGraph (strict)"() -> ("Value"=w422:cluster{"X":sgl[], "Y":sgl[]}, "YScale.NameLbl.Text"=w421:string)  [unwired: 2 in, 2 out]
            n230 = call "Show Data Viewer Plot.vi"("Caption.Text"="TIC Spectrum", "Y Scale.Unit Label.Text"=w421, "Graph"=w422) -> ()  [unwired: 9 in]
          }
        }
      }
      event "Overlays": Mouse Down {
        n231 = event-data() -> ("Mods.Double Click"=w425:bool)  [unwired: 1 out]
        n232 = case shown="True" w425 {
          frame False {
          }
          frame True {
            n233 = local read "Overlays"() -> (w426:cluster{"X":sgl[], "Y":sgl[]}[])
            n234 = call "Show Data Viewer N Plots.vi"("Caption.Text"="Overlays", "Graph"=w426) -> ()  [unwired: 10 in]
          }
        }
      }
    }
  }
